vi "Initialize.vi"(8 "error in":errorcluster, 10 "shared resources":refnum<class "Shared Resources.lvclass">, 11 "Ballard ARINC-429 Tx Execution Unit in":refnum<class "Tx Scheduled Labels Execution Unit.lvclass">) -> (0 "error out":errorcluster, 3 "Ballard ARINC-429 Tx Execution Unit out":refnum<class "Tx Scheduled Labels Execution Unit.lvclass">)   [LabVIEW 2020, in "AIM ARINC 429 Engine.lvlib" / "Implementation.lvlib" / "Tx Scheduled Labels Execution Unit.lvclass"]
uses:
  Tx Scheduled Labels Execution Unit.lvclass
  Custom Device/Custom Device.lvlib
  Execution Unit/Execution Unit.lvclass
  Shared Resources/Shared Resources.lvclass
  C:/Users/nitest/Documents/LabVIEW Data/AIM ARINC 429/Source/Custom Device Support/Engine/Implementation/Execution Unit/Execution Unit.lvclass
  Interfaces/Shared Resources/Shared Resources.lvclass
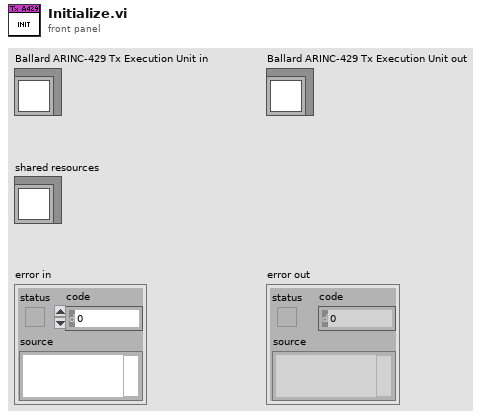
[diagram p1: front panel]
types:
  T1 = typedef "AIM ARINC 429 Engine.lvlib/Custom Device.lvlib/Hardware Handles.ctl" = cluster{"module":u8}
  T2 = typedef "RT Hardware Channel Settings.ctl" = cluster{"channel #":u16, "channel handle":u64, "labels settings for RT":T3[]}
  T3 = typedef "RT Label Settings.ctl" = cluster{"Name":string, "xmlName":string, "label":T4, "transfer period":u32, "SDI_Enabled":bool, "SDI":u8, "parameter driver data":T5, "transfer type":T9, "has timestamp?":bool, "Label Disable/Trigger Channel Reference":T8, "Message Handle":u64, "Initialized?":bool, "Word Initial Raw Value":u32, "Label Timestamp Channel Data Reference":T10, "disabled":bool}
  T4 = typedef "Label.ctl" = u8
  T5 = typedef "RT Parameters.ctl" = cluster{"parameter definitions":T6[], "Tx parameter refs":T8[]}
  T6 = typedef "Parameter Definition.ctl" = cluster{"start index":i32, "size":i32, "encoding":T7, "signed":bool, "scale multiplier":dbl, "scale offset":dbl}
  T7 = typedef "Encoding and Decoding.lvlib/Encoding.ctl" = enum16{"BNR", "BCD", "Discrete"}
  T8 = typedef "Custom Device API.lvlib/Custom Device Item Ref.ctl" = u64
  T9 = typedef "Transfer Type.ctl" = enum16{"Scheduled", "Acyclic", "Block", "Strobe"}
  T10 = typedef "Custom Device API.lvlib/Data Reference.ctl" = i32
  T11 = typedef "Map of Values Indexes to Channel and Label Indexes.ctl" = map{i32, cluster{"channel index":i32, "label index":i32, "group values start index":i32, "values in group":i32}}
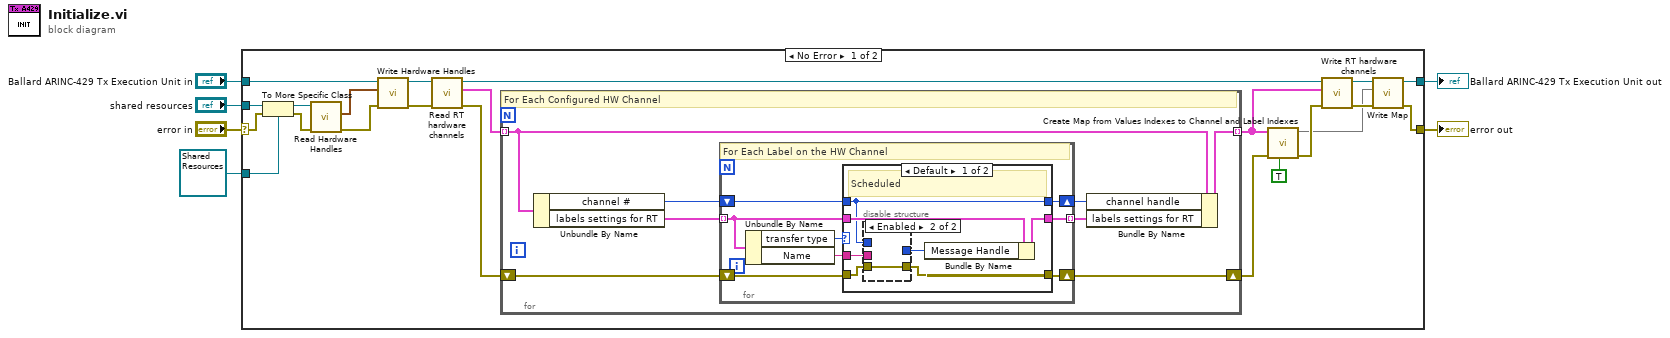
[diagram p0: block diagram]
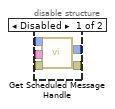
[diagram p2: hidden frame]
diagram:
  n1 = case shown="No Error" "error in" {
    selector: "error in" -> [w12 w61]
    tunnel: "Ballard ARINC-429 Tx Execution Unit in" -> [w16 w62]
    tunnel: [w20 w62] -> w5
    tunnel: [w19 w61] -> w3
    tunnel: "shared resources" -> [w10 _]
    tunnel: refnum<class "Shared Resources.lvclass"> refnum ("Ballard ARINC-429 shared resources in") -> [w9 _]
    frame No Error {
      n2 = To More Specific Class(target class=w9, reference=w10, error in=w12) -> (specific class reference=w8:refnum<class "Shared Resources.lvclass">, error out=w11:errorcluster)
      n3 = call "Read Hardware Handles.vi"("error in"=w11, "Ballard ARINC-429 shared resources in"=w8) -> ("error out"=w17:errorcluster, "hardware handles"=w14:T1)  [unwired: 7 in, 1 out]
      n4 = call "Write Hardware Handles.vi"("error in"=w17, "hardware handles"=w14, "Ballard ARINC-429 Execution Unit in"=w16) -> ("error out"=w13:errorcluster, "Ballard ARINC-429 Execution Unit out"=w15:refnum<class "Tx Scheduled Labels Execution Unit.lvclass">)  [unwired: 7 in]
      n5 = call "Read RT hardware channels.vi"("error in"=w13, "Ballard ARINC-429 Tx Execution Unit in"=w15) -> ("error out"=w26:errorcluster, "RT hardware channels"=w28:T2[], "Ballard ARINC-429 Tx Execution Unit out"=w27:refnum<class "Tx Scheduled Labels Execution Unit.lvclass">)  [unwired: 7 in]
      n6 = for {
        shift-right: [w31] -> w24
        shift-left: w26 -> [w35]
        tunnel: w28 -> [w34] mode=indexing
        tunnel: [w32] -> w25 mode=indexing
        # "For Each Configured HW Channel"
        n7 = Unbundle By Name(w34) -> ("channel #"=w30:u16, "labels settings for RT"=w36:T3[])
        n8 = for {
          tunnel: w36 -> [w39] mode=indexing
          shift-right: [w40] -> w31
          shift-left: w35 -> [w41]
          tunnel: [w38] -> w33 mode=indexing
          shift-right: [w37] -> w29
          shift-left: w30 -> [w43]
          # "For Each Label on the HW Channel"
          n9 = Unbundle By Name(w39) -> ("transfer type"=w44:T9, "Name"=w42:string)
          n10 = case shown="Default" w44 {
            tunnel: w43 -> [w45 w58]
            tunnel: w42 -> [w51 _]
            tunnel: w41 -> [w50 w60]
            tunnel: [w49 w60] -> w40
            tunnel: w39 -> [w47 w59]
            tunnel: [w46 w59] -> w38
            tunnel: [w45 w58] -> w37
            frame Default {
              # "Scheduled"
              n11 = disable-structure shown="Enabled" {
                disable-tunnel: w51 -> [w56 _]
                disable-tunnel: w50 -> [w55 w57]
                disable-tunnel: [w54 w57] -> w49
                disable-tunnel: [w53 _] -> w48
                disable-tunnel: w45 -> [w52 _]
                frame Disabled {
                  n12 = call <instrlib>:"Get Scheduled Message Handle.vi"("error in (no error)"=w55, "message name"=w56, "channel handle in"=w52) -> ("error out"=w54:errorcluster, "message handle out"=w53:u64)  [unwired: 6 in, 1 out]
                }
                frame Enabled {
                }
              }
              n13 = Bundle By Name(cluster=w47, "Message Handle"=w48) -> (w46:T3)
            }
            frame "Acyclic" {
            }
          }
        }
        n14 = Bundle By Name(cluster=w34, "channel handle"=w29, "labels settings for RT"=w33) -> (w32:T2)
      }
      n15 = call "Create Map from Values Indexes to Channel and Label Indexes.vi"("disable channel included in group"=TRUE, "error in"=w24, "RT hardware channels"=w25) -> ("error out"=w23:errorcluster, "map from values index to RT info indexes"=w18:T11)  [unwired: 7 in]
      n16 = call "Write RT hardware channels.vi"("error in"=w23, "RT hardware channels"=w25, "Ballard ARINC-429 Tx Execution Unit in"=w27) -> ("error out"=w22:errorcluster, "Ballard ARINC-429 Tx Execution Unit out"=w21:refnum<class "Tx Scheduled Labels Execution Unit.lvclass">)  [unwired: 7 in]
      n17 = call "Write Map.vi"("error in"=w22, "map from values indexes to RT info indexes"=w18, "Ballard ARINC-429 Tx Execution Unit in"=w21) -> ("error out"=w19:errorcluster, "Ballard ARINC-429 Tx Execution Unit out"=w20:refnum<class "Tx Scheduled Labels Execution Unit.lvclass">)  [unwired: 7 in]
    }
    frame Error {
    }
  }
  "error out" <- w3
  "Ballard ARINC-429 Tx Execution Unit out" <- w5
